vi "Form GGA Sentence.vi"(8 "error in (no error)":errorcluster, 11 "GGA data":T1={"time of fix"={"included?"=TRUE, "time"=timestamp(1451718000 s since 1904-01-01)}, "latitude"={"included?"=TRUE, "latitude (deg)"=0.0}, "longitude"={"included?"=TRUE, "longitude (deg)"=0.0}, "fix quality"={"included?"=TRUE, "quality"=0}, "number of satellites in view"={"included?"=TRUE, "number of satellites"=0}, "horizontal dilution of precision"={"included?"=TRUE, "horizontal DOP"=0.0}, "altitude above mean sea level"={"included?"=TRUE, "altitude (m)"=0.0}, "height of geoid above WGS84"={"included?"=TRUE, "height of geoid (m)"=0.0}, "time since last DGPS update"={"included?"=TRUE, "time (s)"=0.0}, "DGPS station ID number"={"included?"=TRUE, "station ID number"=0.0}} {"fix quality"."quality" items=["Invalid", "GPS Fix", "DGPS Fix", "PPS Fix", "Real Time Kinematic", "Float RTK", "Estimated", "Manual Input Mode", "Simulation Mode"]}) -> (0 "error out":errorcluster, 3 "GGA sentence":string)   [LabVIEW 2011, in "u-blox 5 Series.lvlib"]
doc: "Creates an NMEA sentence using the data you specify for a particular sentence type. You must manually select the polymorphic instance to use."
uses:
  u-blox 5 Series.lvlib
  typedefs/GGA Data.ctl
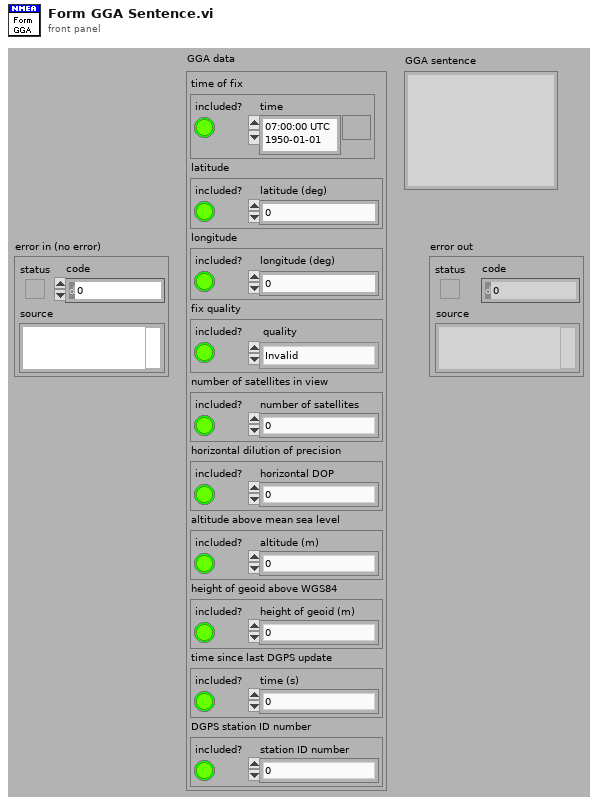
[diagram p1: front panel]
types:
  T1 = typedef "u-blox 5 Series.lvlib/GGA Data.ctl" = cluster{"time of fix":cluster{"included?":bool, "time":timestamp}, "latitude":cluster{"included?":bool, "latitude (deg)":dbl}, "longitude":cluster{"included?":bool, "longitude (deg)":dbl}, "fix quality":cluster{"included?":bool, "quality":u16}, "number of satellites in view":cluster{"included?":bool, "number of satellites":i8}, "horizontal dilution of precision":cluster{"included?":bool, "horizontal DOP":dbl}, "altitude above mean sea level":cluster{"included?":bool, "altitude (m)":dbl}, "height of geoid above WGS84":cluster{"included?":bool, "height of geoid (m)":dbl}, "time since last DGPS update":cluster{"included?":bool, "time (s)":dbl}, "DGPS station ID number":cluster{"included?":bool, "station ID number":dbl}}
  T2 = cluster{"included?":bool, "number of satellites":i8}
  T3 = cluster{"included?":bool, "height of geoid (m)":dbl}
  T4 = cluster{"included?":bool, "station ID number":dbl}
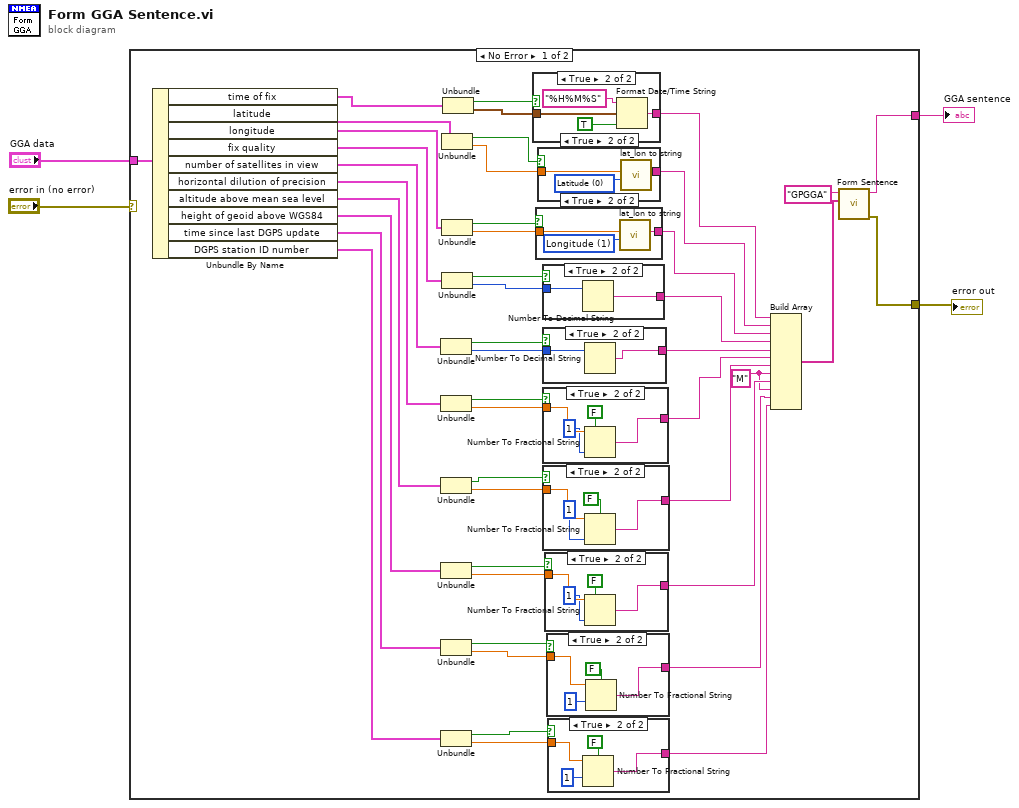
[diagram p0: block diagram]
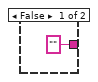
[diagram p2: hidden frame]
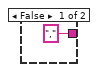
[diagram p3: hidden frame]
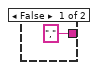
[diagram p4: hidden frame]
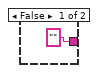
[diagram p5: hidden frame]
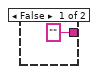
[diagram p6: hidden frame]
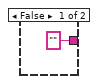
[diagram p7: hidden frame]
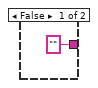
[diagram p8: hidden frame]
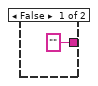
[diagram p9: hidden frame]
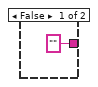
[diagram p10: hidden frame]
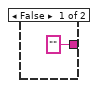
[diagram p11: hidden frame]
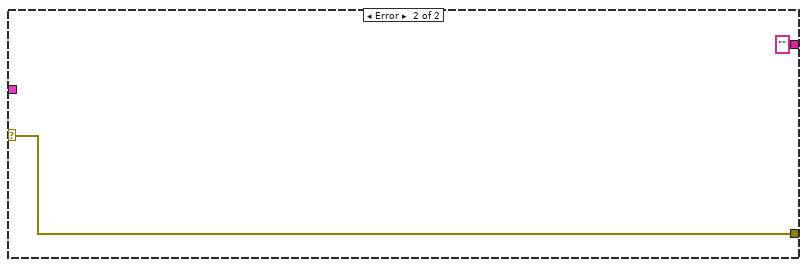
[diagram p12: hidden frame]
diagram:
  n1 = case shown="No Error" "error in (no error)" {
    selector: "error in (no error)" -> [_ w95]
    tunnel: [w49 w95] -> w1
    tunnel: [w48 "" ("NMEA Sentence")] -> w2
    tunnel: "GGA data" -> [w47 _]
    frame No Error {
      w37 = "M" ("element")
      n2 = Unbundle By Name(w47) -> ("time of fix"=w34:cluster{"included?":bool, "time":timestamp}, "latitude"=w32:cluster{"included?":bool, "latitude (deg)":dbl}, "longitude"=w16:cluster{"included?":bool, "longitude (deg)":dbl}, "fix quality"=w18:cluster{"included?":bool, "quality":u16}, "number of satellites in view"=w20:T2, "horizontal dilution of precision"=w22:cluster{"included?":bool, "horizontal DOP":dbl}, "altitude above mean sea level"=w24:cluster{"included?":bool, "altitude (m)":dbl}, "height of geoid above WGS84"=w26:T3, "time since last DGPS update"=w28:cluster{"included?":bool, "time (s)":dbl}, "DGPS station ID number"=w30:T4)
      n3 = Unbundle(w20) -> ("included?"=w9:bool, "number of satellites"=w19:i8)
      n4 = Unbundle(w22) -> ("included?"=w10:bool, "horizontal DOP"=w21:dbl)
      n5 = Unbundle(w24) -> ("included?"=w11:bool, "altitude (m)"=w23:dbl)
      n6 = Unbundle(w26) -> ("included?"=w12:bool, "height of geoid (m)"=w25:dbl)
      n7 = Unbundle(w28) -> ("included?"=w13:bool, "time (s)"=w27:dbl)
      n8 = Unbundle(w30) -> ("included?"=w14:bool, "station ID number"=w29:dbl)
      n9 = Unbundle(w32) -> ("included?"=w5:bool, "latitude (deg)"=w31:dbl)
      n10 = Unbundle(w16) -> ("included?"=w7:bool, "longitude (deg)"=w15:dbl)
      n11 = Unbundle(w18) -> ("included?"=w8:bool, "quality"=w17:u16)
      n12 = Unbundle(w34) -> ("included?"=w6:bool, "time"=w33:timestamp)
      n13 = case shown="True" w6 {
        tunnel: ["" ("date/time string") w54] -> w46
        tunnel: w33 -> [_ w53]
        frame False {
        }
        frame True {
          n14 = Format Date/Time String(time format string (%c)="%H%M%S", seconds (now)=w53, UTC format=TRUE) -> (date/time string=w54:string)
        }
      }
      n15 = case shown="True" w7 {
        tunnel: ["," ("NMEA String for Lat/Lon") w62] -> w45
        tunnel: w15 -> [_ w61]
        frame False {
        }
        frame True {
          w63 = u16 1 items=["Latitude", "Longitude"] ("Lat/Lon")
          n16 = call "lat_lon to string.vi"("lat/lon"=w63, "composite value"=w61) -> ("NMEA string for lat/lon"=w62:string)  [unwired: 9 out]
        }
      }
      n17 = case shown="True" w5 {
        tunnel: ["," ("NMEA String for Lat/Lon") w58] -> w41
        tunnel: w31 -> [_ w57]
        frame False {
        }
        frame True {
          w59 = u16 0 items=["Latitude", "Longitude"] ("Lat/Lon")
          n18 = call "lat_lon to string.vi"("lat/lon"=w59, "composite value"=w57) -> ("NMEA string for lat/lon"=w58:string)  [unwired: 9 out]
        }
      }
      n19 = case shown="True" w8 {
        tunnel: ["" w66] -> w40
        tunnel: w17 -> [_ w65]
        frame False {
        }
        frame True {
          n20 = Number To Decimal String(number=w65) -> (decimal integer string=w66:string)  [unwired: 1 out]
        }
      }
      n21 = case shown="True" w9 {
        tunnel: ["" w69] -> w44
        tunnel: w19 -> [_ w68]
        frame False {
        }
        frame True {
          n22 = Number To Decimal String(number=w68) -> (decimal integer string=w69:string)  [unwired: 1 out]
        }
      }
      n23 = case shown="True" w10 {
        tunnel: ["" w74] -> w43
        tunnel: w21 -> [_ w73]
        frame False {
        }
        frame True {
          n24 = Number To Fractional String(use system decimal point (T)=FALSE, number=w73, precision (6)=i16 1) -> (F-format string=w74:string)  [unwired: 1 out]
        }
      }
      n25 = case shown="True" w11 {
        tunnel: ["" w79] -> w39
        tunnel: w23 -> [_ w78]
        frame False {
        }
        frame True {
          n26 = Number To Fractional String(use system decimal point (T)=FALSE, number=w78, precision (6)=i16 1) -> (F-format string=w79:string)  [unwired: 1 out]
        }
      }
      n27 = case shown="True" w12 {
        tunnel: ["" w84] -> w38
        tunnel: w25 -> [_ w83]
        frame False {
        }
        frame True {
          n28 = Number To Fractional String(use system decimal point (T)=FALSE, number=w83, precision (6)=i16 1) -> (F-format string=w84:string)  [unwired: 1 out]
        }
      }
      n29 = case shown="True" w13 {
        tunnel: ["" w89] -> w36
        tunnel: w27 -> [_ w88]
        frame False {
        }
        frame True {
          n30 = Number To Fractional String(use system decimal point (T)=FALSE, number=w88, precision (6)=i16 1) -> (F-format string=w89:string)  [unwired: 1 out]
        }
      }
      n31 = case shown="True" w14 {
        tunnel: ["" w94] -> w35
        tunnel: w29 -> [_ w93]
        frame False {
        }
        frame True {
          n32 = Number To Fractional String(use system decimal point (T)=FALSE, number=w93, precision (6)=i16 1) -> (F-format string=w94:string)  [unwired: 1 out]
        }
      }
      n33 = Build Array(w46, w41, w45, w40, w44, w43, w39, w37, w38, w37, w36, w35) -> (w42:string[])
      n34 = call "Form Sentence.vi"("sentence data"=w42, "sentence type"="GPGGA" ("Sentence Type")) -> ("error out"=w49:errorcluster, "sentence"=w48:string)  [unwired: 6 in]
    }
    frame Error {
    }
  }
  "error out" <- w1
  "GGA sentence" <- w2
